vi "Example MQTT Websockets Client-Server.vi"() -> ()   [LabVIEW 2013]
uses:
  <vilib>/LabVIEW Open Source Project/Connection/Connection/Connection.lvclass
  MQTT_Websockets/Connection/WebsocketsConnection.lvclass
panel:
  out "client2 session error":errorcluster
  out "Received Bytes (2)":u8[](array[numeric]) format="%.0b"
  out "value 2":dbl
  out "Comm2 OK":bool
  out "client2 connected":bool
  out "Sent Bytes (2)":u8[](array[numeric]) format="%.0b"
  in  "STOP CLIENT 2":bool
  in  "STOP CLIENT 1":bool
  out "Sent Bytes (1)":u8[](array[numeric]) format="%.0b"
  out "client1 connected":bool
  out "Comm1 OK":bool
  out "value":dbl
  out "client1 session error":errorcluster
  out "Received Bytes (1)":u8[](array[numeric]) format="%.0b"
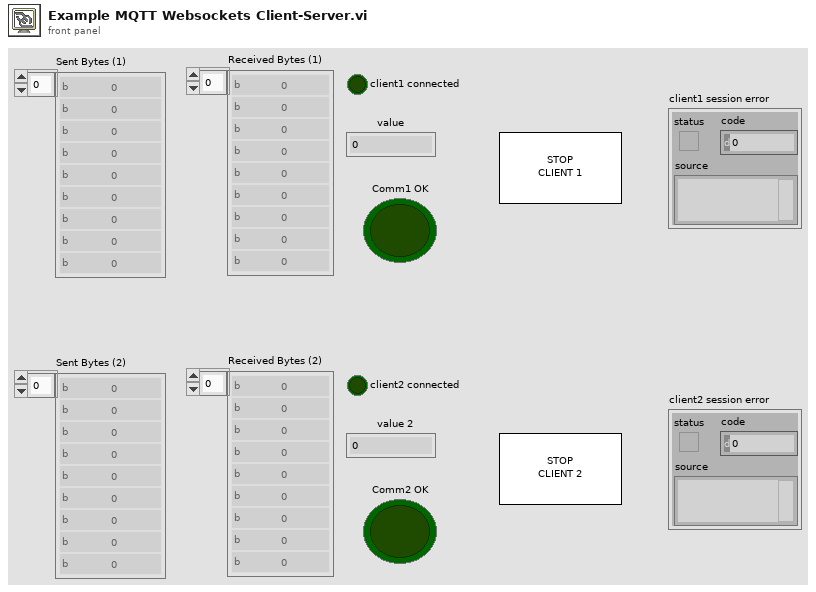
[diagram p1: front panel]
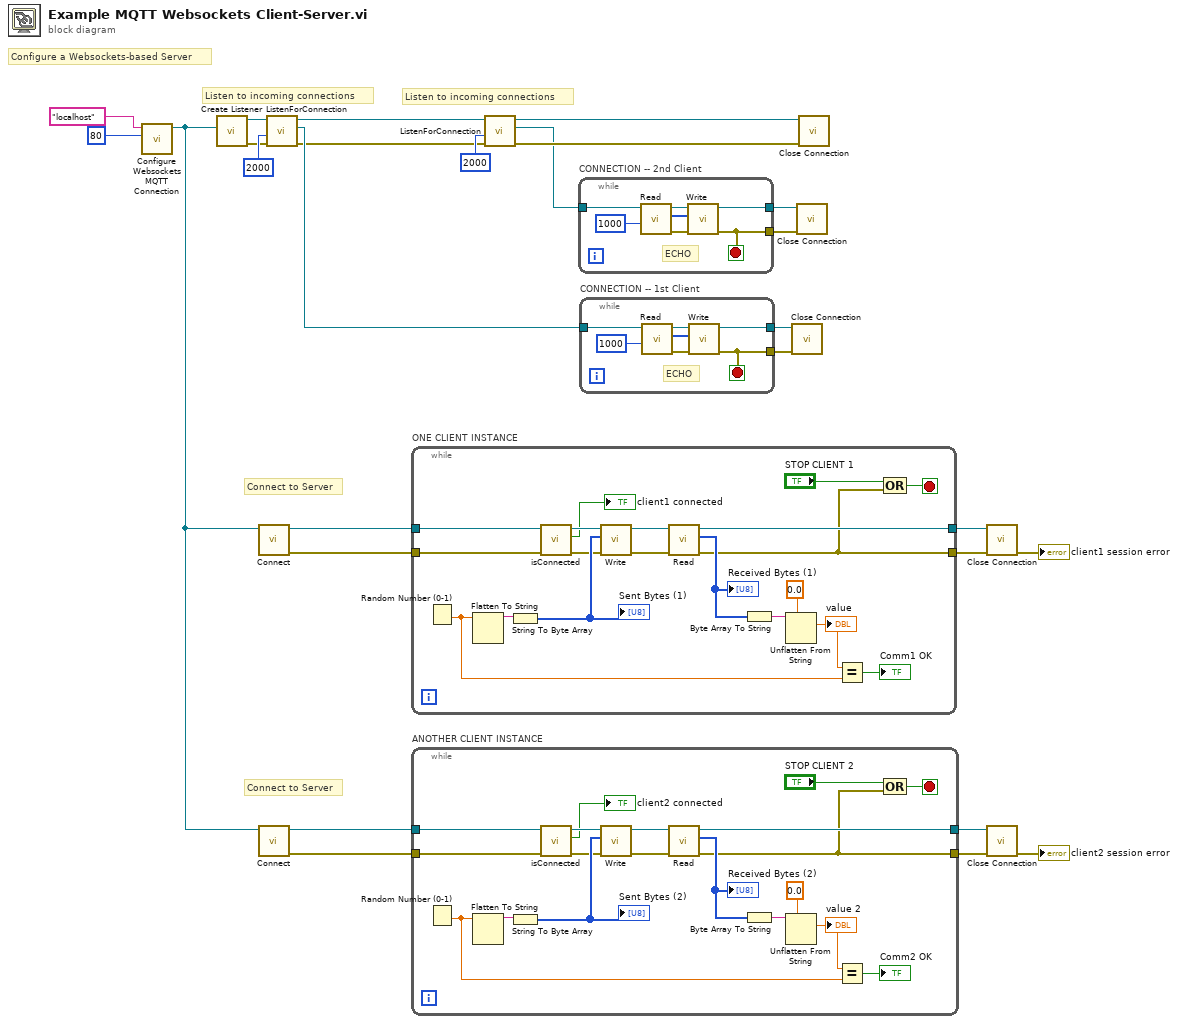
[diagram p0: block diagram]
diagram:
  # "Connect to Server"
  # "Listen to incoming connections"
  # "Connect to Server"
  # "Listen to incoming connections"
  # "Configure a Websockets-based Server"
  n1 = call "Configure Websockets MQTT Connection.vi"("remote port (80)"=u16 80, "address (localhost)"="localhost") -> ("WSConnection"=w1:refnum<class "WebsocketsConnection.lvclass">)  [unwired: 8 in, 1 out]
  n2 = call <vilib>:"Create Listener.vi"("Connection Configuration"=w1) -> ("error out"=w25:errorcluster, "Listener"=w27:refnum<class "WebsocketsConnection.lvclass">)  [unwired: 9 in]
  n3 = call <vilib>:"Connect.vi"("Connection in"=w1) -> ("error out"=w18:errorcluster, "Connection out"=w17:refnum<class "WebsocketsConnection.lvclass">)  [unwired: 9 in]
  n4 = call <vilib>:"Connect.vi"("Connection in"=w1) -> ("error out"=w4:errorcluster, "Connection out"=w5:refnum<class "WebsocketsConnection.lvclass">)  [unwired: 9 in]
  n5 = call <vilib>:"ListenForConnection.vi"("error in (no error)"=w25, "timeout (2000 ms)"=2000 ("bytes to read (100)"), "Listener"=w27) -> ("error out"=w11:errorcluster, "Connection"=w19:refnum<class "Connection.lvclass">, "Listener out"=w13:refnum<class "WebsocketsConnection.lvclass">)  [unwired: 5 in, 1 out]
  n6 = while "ONE CLIENT INSTANCE" {
    tunnel: [w40] -> w22
    tunnel: w18 -> [w36]
    tunnel: w17 -> [w34]
    tunnel: [w29] -> w16
    stop <- w28 stop-if-true
    n7 = Random Number (0-1)() -> (number: 0 to 1=w38:dbl)
    n8 = Flatten To String(anything=w38) -> (data string=w45:string)  [unwired: 3 in, 2 out]
    n9 = String To Byte Array(string=w45) -> (unsigned byte array=w44:u8[])
    "Sent Bytes (1)" <- w44
    n10 = call <vilib>:"isConnected.vi"("error in (no error)"=w36, "Connection in"=w34) -> ("error out"=w35:errorcluster, "connected"=→"client1 connected":bool, "Connection out"=w33:refnum<class "WebsocketsConnection.lvclass">)  [unwired: 7 in]
    n11 = call <vilib>:"Write.vi"("error in (no error)"=w35, "Bytes"=w44, "Connection in"=w33) -> ("error out"=w31:errorcluster, "Connection"=w46:refnum<class "WebsocketsConnection.lvclass">)  [unwired: 7 in]
    n12 = call <vilib>:"Read.vi"("error in (no error)"=w31, "TCPConnection in"=w46) -> ("error out"=w29:errorcluster, "Bytes"=w43:u8[], "TCPConnection out"=w40:refnum<class "WebsocketsConnection.lvclass">)  [unwired: 5 in, 2 out]
    "Received Bytes (1)" <- w43
    n13 = Byte Array To String(unsigned byte array=w43) -> (string=w42:string)
    n14 = Unflatten From String(type=0.0, binary string=w42) -> (value=w39:dbl)  [unwired: 3 in, 2 out]
    "value" <- w39
    n15 = Equal?(x=w39, y=w38) -> (x = y?=→"Comm1 OK":bool)
    n16 = Compound Arithmetic op=OR("STOP CLIENT 1", w29) -> (w28:bool)
  }
  n17 = while "ANOTHER CLIENT INSTANCE" {
    tunnel: [w59] -> w3
    tunnel: w4 -> [w55]
    tunnel: w5 -> [w53]
    tunnel: [w48] -> w6
    stop <- w47 stop-if-true
    n18 = Random Number (0-1)() -> (number: 0 to 1=w57:dbl)
    n19 = Flatten To String(anything=w57) -> (data string=w64:string)  [unwired: 3 in, 2 out]
    n20 = String To Byte Array(string=w64) -> (unsigned byte array=w63:u8[])
    "Sent Bytes (2)" <- w63
    n21 = call <vilib>:"isConnected.vi"("error in (no error)"=w55, "Connection in"=w53) -> ("error out"=w54:errorcluster, "connected"=→"client2 connected":bool, "Connection out"=w52:refnum<class "WebsocketsConnection.lvclass">)  [unwired: 7 in]
    n22 = call <vilib>:"Write.vi"("error in (no error)"=w54, "Bytes"=w63, "Connection in"=w52) -> ("error out"=w50:errorcluster, "Connection"=w65:refnum<class "WebsocketsConnection.lvclass">)  [unwired: 7 in]
    n23 = call <vilib>:"Read.vi"("error in (no error)"=w50, "TCPConnection in"=w65) -> ("error out"=w48:errorcluster, "Bytes"=w62:u8[], "TCPConnection out"=w59:refnum<class "WebsocketsConnection.lvclass">)  [unwired: 5 in, 2 out]
    "Received Bytes (2)" <- w62
    n24 = Byte Array To String(unsigned byte array=w62) -> (string=w61:string)
    n25 = Unflatten From String(type=0.0, binary string=w61) -> (value=w58:dbl)  [unwired: 3 in, 2 out]
    "value 2" <- w58
    n26 = Equal?(x=w58, y=w57) -> (x = y?=→"Comm2 OK":bool)
    n27 = Compound Arithmetic op=OR("STOP CLIENT 2", w48) -> (w47:bool)
  }
  n28 = call <vilib>:"ListenForConnection.vi"("error in (no error)"=w11, "timeout (2000 ms)"=2000 ("bytes to read (100)"), "Listener"=w13) -> ("error out"=w10:errorcluster, "Connection"=w9:refnum<class "Connection.lvclass">, "Listener out"=w12:refnum<class "WebsocketsConnection.lvclass">)  [unwired: 5 in, 1 out]
  n29 = while "CONNECTION -- 2nd Client" {
    tunnel: [w69] -> w7
    tunnel: w9 -> [w66]
    tunnel: [w67] -> w8
    stop <- w67 stop-if-true
    # "ECHO"
    n30 = call <vilib>:"Read.vi"("timeout (2000 ms)"=1000 ("bytes to read (100)"), "TCPConnection in"=w66) -> ("error out"=w70:errorcluster, "Bytes"=w68:u8[], "TCPConnection out"=w71:refnum<class "Connection.lvclass">)  [unwired: 5 in, 2 out]
    n31 = call <vilib>:"Write.vi"("error in (no error)"=w70, "Bytes"=w68, "Connection in"=w71) -> ("error out"=w67:errorcluster, "Connection"=w69:refnum<class "Connection.lvclass">)  [unwired: 7 in]
  }
  n32 = while "CONNECTION -- 1st Client" {
    tunnel: [w76] -> w24
    tunnel: w19 -> [w73]
    tunnel: [w74] -> w15
    stop <- w74 stop-if-true
    # "ECHO"
    n33 = call <vilib>:"Read.vi"("timeout (2000 ms)"=1000 ("bytes to read (100)"), "TCPConnection in"=w73) -> ("error out"=w77:errorcluster, "Bytes"=w75:u8[], "TCPConnection out"=w78:refnum<class "Connection.lvclass">)  [unwired: 5 in, 2 out]
    n34 = call <vilib>:"Write.vi"("error in (no error)"=w77, "Bytes"=w75, "Connection in"=w78) -> ("error out"=w74:errorcluster, "Connection"=w76:refnum<class "Connection.lvclass">)  [unwired: 7 in]
  }
  n35 = call <vilib>:"Close Connection.vi"("error in (no error)"=w15, "Connection in"=w24) -> ()  [unwired: 8 in, 2 out]
  n36 = call <vilib>:"Close Connection.vi"("error in (no error)"=w8, "Connection in"=w7) -> ()  [unwired: 8 in, 2 out]
  n37 = call <vilib>:"Close Connection.vi"("error in (no error)"=w10, "Connection in"=w12) -> ()  [unwired: 8 in, 2 out]
  n38 = call <vilib>:"Close Connection.vi"("error in (no error)"=w16, "Connection in"=w22) -> ("error out"=→"client1 session error":errorcluster)  [unwired: 8 in, 1 out]
  n39 = call <vilib>:"Close Connection.vi"("error in (no error)"=w6, "Connection in"=w3) -> ("error out"=→"client2 session error":errorcluster)  [unwired: 8 in, 1 out]
